vi "SetPersistentConfiguration.vi"(8 "ErrorIn":errorcluster, 9 "DataIn":variant, 11 "ReferenceIn":refnum<class "VerticalButtonBar.lvclass">) -> (0 "ErrorOut":errorcluster, 1 "DataOut":variant, 3 "ReferenceOut":refnum<class "VerticalButtonBar.lvclass">)   [LabVIEW 2021, in "VerticalButtonBar.lvclass"]
uses:
  VerticalButtonBar.lvclass
  a2d9dd7e-4f73-47a2-b010-087cab1955c7.vi
  <vilib>/Utility/LVClass/Get LV Class Name.vi
  .Externals/Library_TAF_ApplicationFramework/TAFBaseGUI/TAFBaseGUI.lvclass
  VerticalButtonBar.lvclass/VerticalButtonBar.ctl
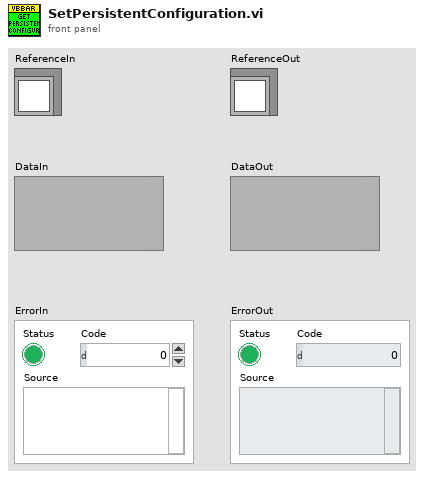
[diagram p1: front panel]
types:
  T1 = typedef "VerticalButtonBar.lvclass/ObjectAttributes.ctl" = cluster{"Interfaces":cluster{"IDockGUI":refnum<class "IDockGUI.lvclass">, "Authorizer":refnum<class "IAuthorization.lvclass">}, "Locals":cluster{"ButtonBar":refnum<class "ButtonCollection.lvclass">, "BaseConfigurationPath":path, "Labels":cluster{"Label":string, "Value":string}[]}, "Persistent":cluster{"ButtonDefinitionFile":string}}
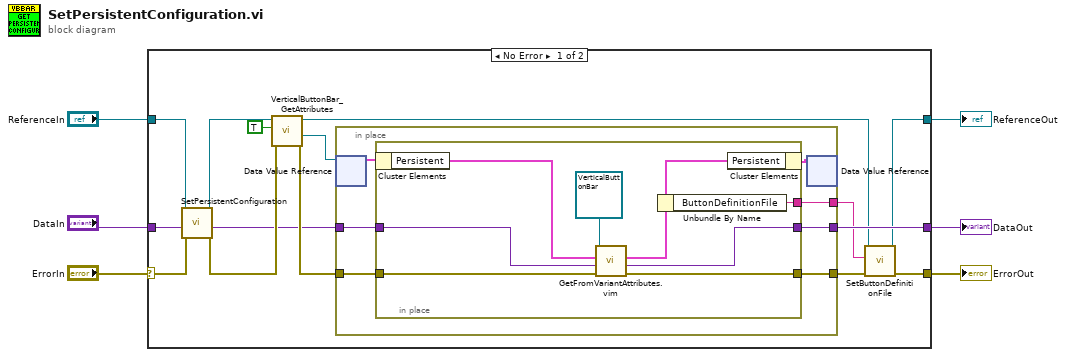
[diagram p0: block diagram]
diagram:
  n1 = case shown="No Error" "ErrorIn" {
    selector: "ErrorIn" -> [w19 w39]
    tunnel: [w17 w39] -> w5
    tunnel: [w8 w38] -> w3
    tunnel: "ReferenceIn" -> [w10 w38]
    tunnel: [w16 w37] -> w2
    tunnel: "DataIn" -> [w12 w37]
    frame No Error {
      n2 = call-parent "SetPersistentConfiguration.vi"("ErrorIn"=w19, "DataIn"=w12, "ReferenceIn"=w10) -> ("ErrorOut"=w18:errorcluster, "DataOut"=w13:variant, "ReferenceOut"=w11:refnum<class "VerticalButtonBar.lvclass">)  [unwired: 6 in]
      n3 = call "VerticalButtonBar_GetAttributes.vi"("ErrorIn"=w18, "OnlyGetDvrReference(False)"=TRUE, "ReferenceIn"=w11) -> ("ErrorOut"=w21:errorcluster, "DataRef"=w14:refnum<data-value>, "ReferenceOut"=w9:refnum<class "VerticalButtonBar.lvclass">)  [unwired: 5 in, 1 out]
      n4 = in-place {
        in-place-border: w21 -> [w28]
        in-place-border: [w27] -> w20
        in-place-border: w13 -> [w26]
        in-place-border: [w25] -> w16
        in-place-border: [w22] -> w7
        n5 = in-place-dvr #1(w14) -> (w24:T1)  [unwired: 1 out]
        n6 = in-place {
          in-place-border: w28 -> [w36]
          in-place-border: [w35] -> w27
          in-place-border: w26 -> [w34]
          in-place-border: [w33] -> w25
          in-place-border: [w29] -> w22
          n7 = in-place-cluster #2(w24) -> ("Persistent"=w31:cluster{"ButtonDefinitionFile":string})
          n8 = call "GetFromVariantAttributes.vim"("ErrorIn"=w36, "DataInIn"=w34, "PersistentDataType"=w31, "Object"=refnum<class "VerticalButtonBar.lvclass"> refnum ("VerticalButtonBar")) -> ("ErrorOut"=w35:errorcluster, "DataOut"=w33:variant, "PersistentDataOut"=w30:cluster{"ButtonDefinitionFile":string})  [unwired: 5 in]
          n9 = Unbundle By Name(w30) -> ("ButtonDefinitionFile"=w29:string)
          n10 = in-place-cluster #2("Persistent"=w30) -> (w23:T1)
        }
        n11 = in-place-dvr #1(w23) -> ()  [unwired: 2 out]
      }
      n12 = call-dynamic "SetButtonDefinitionFile.vi"("ErrorIn"=w20, "ButtonDefinitionFile"=w7, "ReferenceIn"=w9) -> ("ErrorOut"=w17:errorcluster, "ReferenceIn"=w8:refnum<class "VerticalButtonBar.lvclass">)  [unwired: 7 in]
    }
    frame Error {
    }
  }
  "ErrorOut" <- w5
  "ReferenceOut" <- w3
  "DataOut" <- w2
